vi "Get Package Path.vi"() -> ()   [LabVIEW 2021]
panel:
  out "return value":string
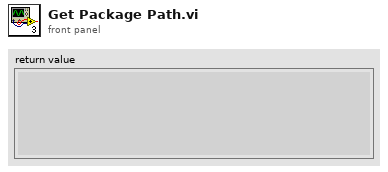
[diagram p1: front panel]
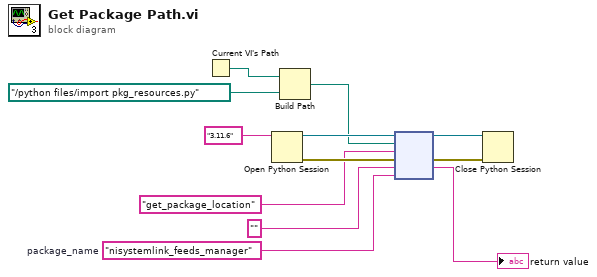
[diagram p0: block diagram]
diagram:
  w8 = "nisystemlink_feeds_manager"  # package_name
  n1 = Current VI's Path() -> (path=w3:path)
  n2 = Open Python Session(python version="3.11.6" ("Python version")) -> (session out=w11:refnum<k35>, error out=w10:errorcluster)  [unwired: 2 in]
  n3 = Build Path(base path=w3, name or relative path=path "../python files/import pkg_resources.py") -> (appended path=w1:path)
  n4 = node(w11, w1, "get_package_location" ("Python version"), w10, "", w8) -> (w5:refnum<k35>, w6:errorcluster, →"return value":string)  [unwired: 1 in, 2 out]
  n5 = Close Python Session(session in=w5, error in=w6) -> ()  [unwired: 1 out]
